vi "Fluids #4.vi"() -> ()   [LabVIEW 2017]
uses:
  <vilib>/addons/control/pid/pid.llb/PID Control Input Filter (DBL).vi
  <vilib>/addons/control/pid/pid.llb/PID Advanced (DBL).vi
  <vilib>/addons/control/pid/NI_PID_pid.lvlib
panel:
  in  "stop":bool
  in  "Pump Switch":bool
  out "Pump Delta P":dbl format="%.1f"
  out "Globe Valve Delta P":dbl format="%.1f"
  out "Ball Valve Delta P":dbl format="%.1f"
  out "EL Delta P":dbl format="%.1f"
  out "TEE Delta P":dbl format="%.1f"
  out "Pipe Delta P":dbl format="%.1f"
  out "U Delta P":dbl format="%.1f"
  out "Fluid Temperature":dbl=19.966648625034704 format="%.1f"
  in  "Flowrate Setpoint":dbl=10.0 caption="gal/min" format="%.1f"
  out "Liquid Flowrate":dbl=-2.4682881675745557e-11 format="%.1f"
  out "Control Valve":dbl(slide)=100.0 scale=0.0..100.0
  in  "Manual Control Override":bool=TRUE
  in  "Set Manual Valve Position":dbl(slide)=100.0 scale=0.0..100.0
  in  "Kc":dbl=2.0
  in  "Ti":dbl=0.05 caption="(min)"
  in  "Td":dbl caption="(min)"
  in  "Main Power":bool
  in  "Pump Speed Setpoint":dbl=100.0 caption="% of Nominal (3450 rpm)" min=0.0 max=125.0 format="%#.1f"
  out "Actual Pump Speed":dbl caption="RPM" format="%#.0f"
  out "Bypass Flowrate":dbl caption="gal/min" format="%#.1f"
  out "Bypass Delta P":dbl caption="psi" format="%#.1g"
  out "Pump Motor Power":dbl caption="W" format="%#.0f"
  out "Control Valve Delta P":dbl caption="psi" format="%#.1g"
  out "Data Point Count":i32
  in  "Specify Time between Data Points (sec)":dbl=1.0
  in  "Cancel Data Collection":bool
  in  "Specify number of data points":i16=1
  in  "Enable 3":bool
  out "Saving Data 3":bool
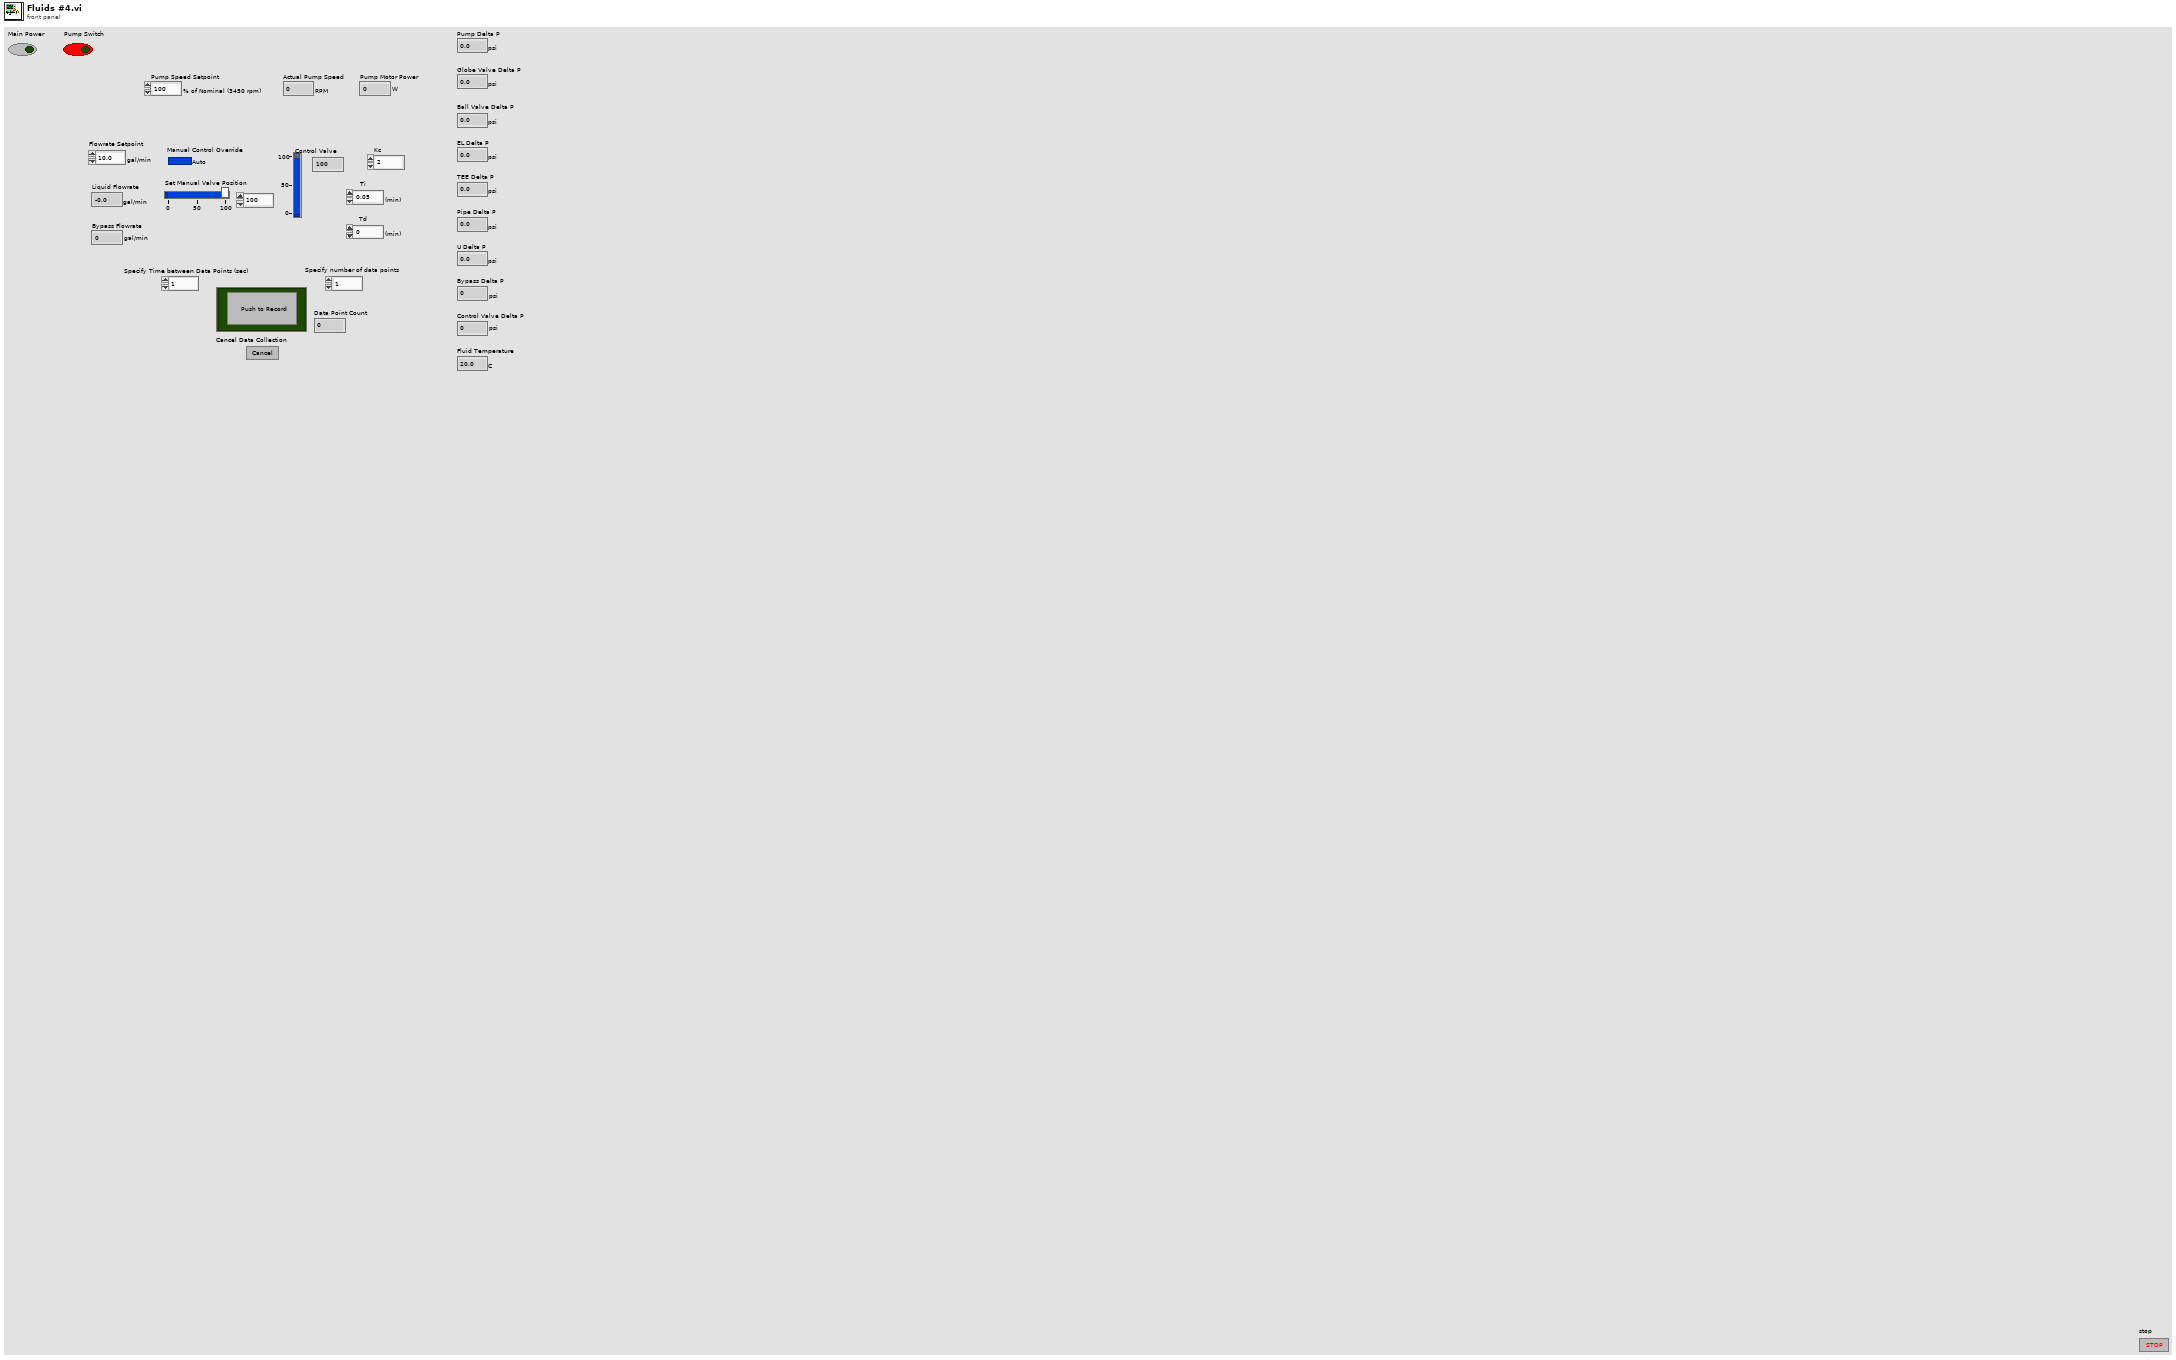
[diagram p1: front panel]
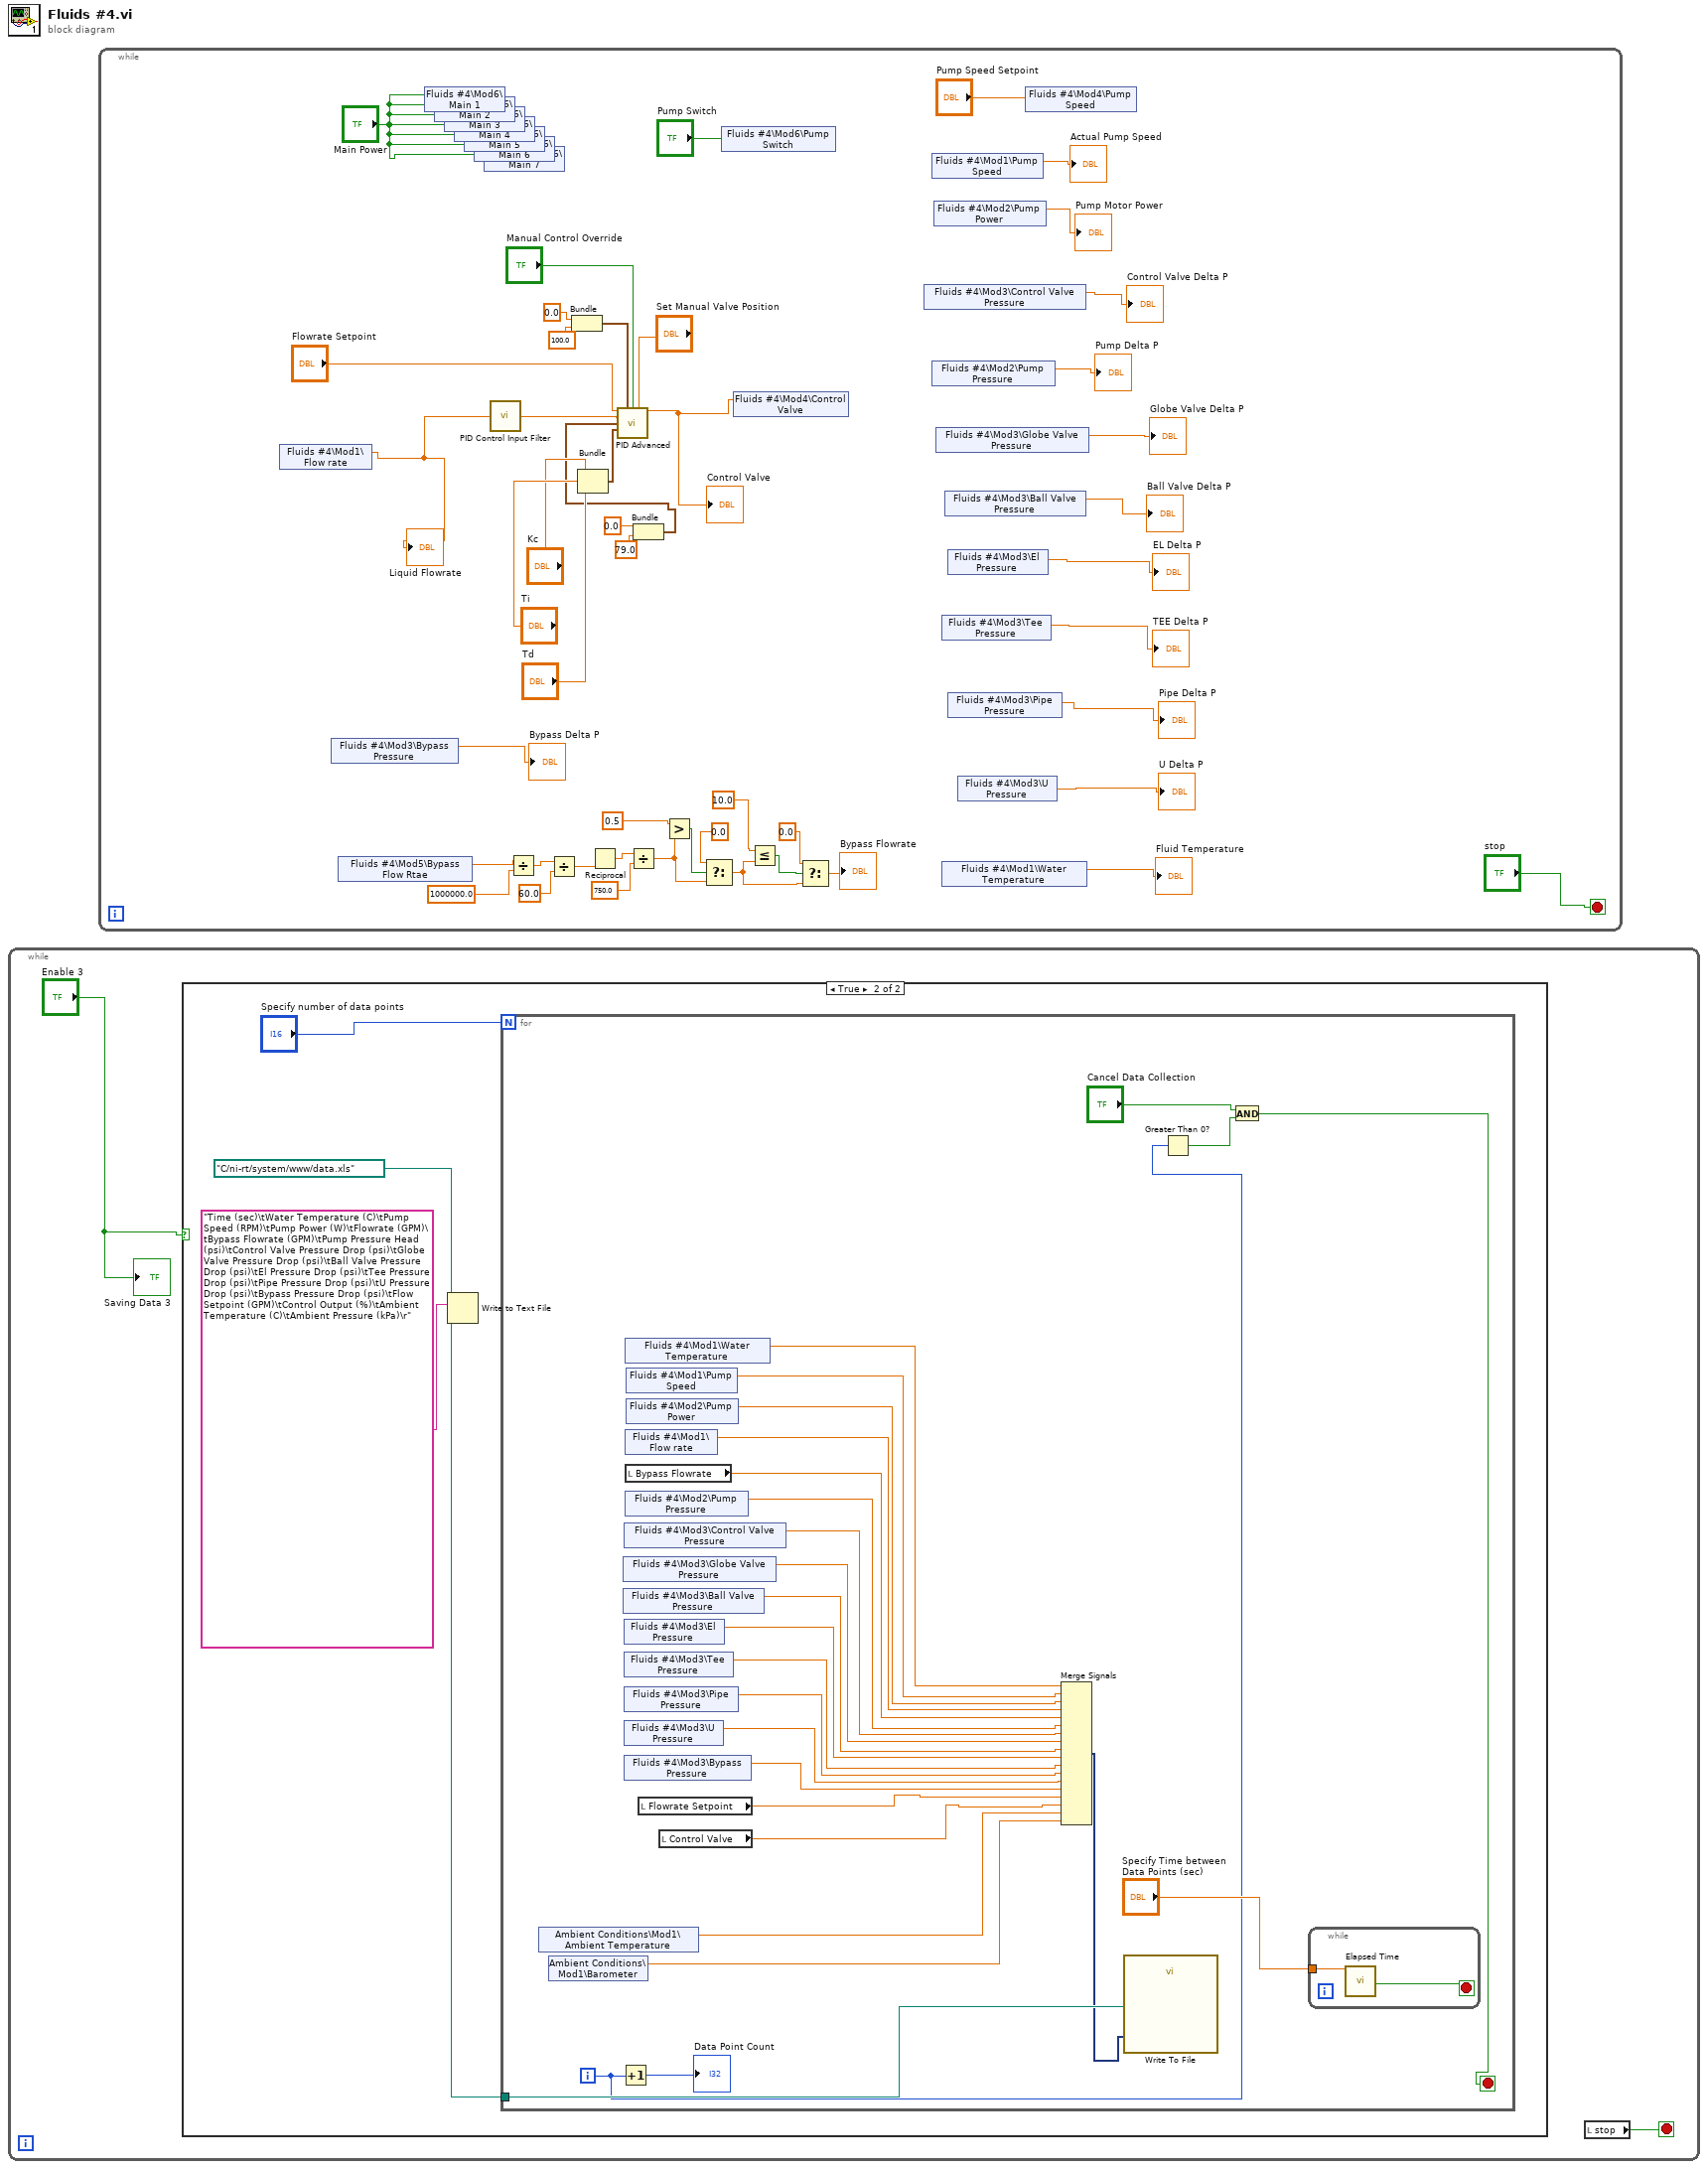
[diagram p0: block diagram]
diagram:
  n1 = while {
    stop <- w1 stop-if-true
    n2 = case shown="True" "Enable 3" {
      frame False {
      }
      frame True {
        w4 = path "C:/ni-rt/system/www/data.xls" ("Filename")
        n3 = Write to Text File(file (use dialog)=w4, text="Time (sec)\tWater Temperature (C)\tPump Speed (RPM)\tPump Power (W)\tFlowrate (GPM)\tBypass Flowrate (GPM)\tPump Pressure Head (psi)\tControl Valve Pressure Drop (psi)\tGlobe Valve Pressure Drop (psi)\tBall Valve Pressure Drop (psi)\tEl Pressure Drop (psi)\tTee Pressure Drop (psi)\tPipe Pressure Drop (psi)\tU Pressure Drop (psi)\tBypass Pressure Drop (psi)\tFlow Setpoint (GPM)\tControl Output (%)\tAmbient Temperature (C)\tAmbient Pressure (kPa)\r") -> ()  [unwired: 2 in, 3 out]
        n4 = for {
          N: "Specify number of data points" -> [_]
          tunnel: w4 -> [w31]
          i -> [w27]
          stop <- w24 stop-if-true
          n5 = shared-variable "Ambient Conditions\\Mod1\\Ambient Temperature"() -> (w23:dbl)  [unwired: 1 in, 1 out]
          n6 = shared-variable "Ambient Conditions\\Mod1\\Barometer"() -> (w22:dbl)  [unwired: 1 in, 1 out]
          n7 = Increment(x=w27) -> (x+1=→"Data Point Count":i32)
          n8 = shared-variable "Fluids #4\\Mod3\\Globe Valve Pressure"() -> (w15:dbl)  [unwired: 1 in, 1 out]
          n9 = shared-variable "Fluids #4\\Mod3\\Ball Valve Pressure"() -> (w16:dbl)  [unwired: 1 in, 1 out]
          n10 = shared-variable "Fluids #4\\Mod3\\Control Valve Pressure"() -> (w14:dbl)  [unwired: 1 in, 1 out]
          n11 = shared-variable "Fluids #4\\Mod3\\El Pressure"() -> (w17:dbl)  [unwired: 1 in, 1 out]
          n12 = shared-variable "Fluids #4\\Mod3\\Tee Pressure"() -> (w18:dbl)  [unwired: 1 in, 1 out]
          n13 = shared-variable "Fluids #4\\Mod3\\Pipe Pressure"() -> (w19:dbl)  [unwired: 1 in, 1 out]
          n14 = shared-variable "Fluids #4\\Mod3\\U Pressure"() -> (w20:dbl)  [unwired: 1 in, 1 out]
          n15 = shared-variable "Fluids #4\\Mod3\\Bypass Pressure"() -> (w21:dbl)  [unwired: 1 in, 1 out]
          n16 = shared-variable "Fluids #4\\Mod1\\Water Temperature"() -> (w9:dbl)  [unwired: 1 in, 1 out]
          n17 = shared-variable "Fluids #4\\Mod1\\Flow rate"() -> (w12:dbl)  [unwired: 1 in, 1 out]
          n18 = local read "Bypass Flowrate"() -> (w6:dbl)
          n19 = shared-variable "Fluids #4\\Mod2\\Pump Pressure"() -> (w13:dbl)  [unwired: 1 in, 1 out]
          n20 = shared-variable "Fluids #4\\Mod1\\Pump Speed"() -> (w10:dbl)  [unwired: 1 in, 1 out]
          n21 = shared-variable "Fluids #4\\Mod2\\Pump Power"() -> (w11:dbl)  [unwired: 1 in, 1 out]
          n22 = local read "Flowrate Setpoint"() -> (w8:dbl)
          n23 = local read "Control Valve"() -> (w7:dbl)
          n24 = Merge Signals(w9, w10, w11, w12, w6, w13, w14, w15, w16, w17, w18, w19, w20, w21, w8, w7, w23, w22) -> (w29:dynamicdata)
          n25 = call "Write To File"("Signals"=w29, "Filename"=w31) -> ()  [unwired: 15 in, 3 out]
          n26 = Greater Than 0?(x=w27) -> (x > 0?=w25:bool)
          n27 = And(x="Cancel Data Collection", y=w25) -> (x .and. y?=w24:bool)
          n28 = while {
            tunnel: "Specify Time between Data Points (sec)" -> [w32]
            stop <- w33 stop-if-true
            n29 = call "Elapsed Time"("Time Target (s)"=w32) -> ("Time has Elapsed"=w33:bool)  [unwired: 11 in, 7 out]
          }
        }
      }
    }
    n30 = local read "stop"() -> (w1:bool)
    "Saving Data 3" <- "Enable 3"
  }
  n31 = while {
    stop <- "stop" stop-if-true
    n32 = shared-variable "Fluids #4\\Mod1\\Flow rate"() -> (w62:dbl)  [unwired: 1 in, 1 out]
    "Liquid Flowrate" <- w62
    n33 = shared-variable "Fluids #4\\Mod3\\Bypass Pressure"() -> (→"Bypass Delta P":dbl)  [unwired: 1 in, 1 out]
    n34 = shared-variable "Fluids #4\\Mod5\\Bypass Flow Rtae"() -> (w52:dbl)  [unwired: 1 in, 1 out]
    n35 = shared-variable "Fluids #4\\Mod6\\Main 1"("Main Power") -> ()  [unwired: 1 in, 1 out]
    n36 = shared-variable "Fluids #4\\Mod6\\Main 2"("Main Power") -> ()  [unwired: 1 in, 1 out]
    n37 = shared-variable "Fluids #4\\Mod6\\Main 3"("Main Power") -> ()  [unwired: 1 in, 1 out]
    n38 = shared-variable "Fluids #4\\Mod6\\Main 4"("Main Power") -> ()  [unwired: 1 in, 1 out]
    n39 = shared-variable "Fluids #4\\Mod6\\Main 5"("Main Power") -> ()  [unwired: 1 in, 1 out]
    n40 = shared-variable "Fluids #4\\Mod6\\Main 6"("Main Power") -> ()  [unwired: 1 in, 1 out]
    n41 = shared-variable "Fluids #4\\Mod6\\Main 7"("Main Power") -> ()  [unwired: 1 in, 1 out]
    n42 = call-poly <vilib>:"PID Control Input Filter.vi"("input"=w62) -> ("output"=w68:dbl)  [unwired: 4 in]
    n43 = Divide(x=w52, y=1000000.0) -> (x/y=w50:dbl)
    n44 = Divide(x=w50, y=60.0) -> (x/y=w48:dbl)
    n45 = Bundle(0.0, 100.0) -> (w70:cluster{dbl, dbl})  [unwired: 1 in]
    n46 = Bundle("Kc"="Kc", "Ti"="Ti", "Td"="Td") -> (w80:cluster{"Kc":dbl, "Ti":dbl, "Td":dbl})  [unwired: 1 in]
    n47 = Reciprocal(x=w48) -> (1/x=w47:dbl)
    n48 = Divide(x=w47, y=750.0) -> (x/y=w44:dbl)
    n49 = Bundle(0.0, 79.0) -> (w74:cluster{dbl, dbl})  [unwired: 1 in]
    n50 = call-poly <vilib>:"PID Advanced.vi"("setpoint"="Flowrate Setpoint", "output range"=w70, "auto? (T)"="Manual Control Override", "manual control"="Set Manual Valve Position", "process variable"=w68, "setpoint range"=w74, "PID gains"=w80) -> ("output"=w35:dbl)  [unwired: 7 in, 1 out]
    "Control Valve" <- w35
    n51 = Greater?(x=0.5, y=w44) -> (0:w42:bool)
    n52 = Select(t=0.0, s=w42, f=w44) -> (s? t:f=w41:dbl)
    n53 = shared-variable "Fluids #4\\Mod6\\Pump Switch"("Pump Switch") -> ()  [unwired: 1 in, 1 out]
    n54 = shared-variable "Fluids #4\\Mod4\\Control Valve"(w35) -> ()  [unwired: 1 in, 1 out]
    n55 = Less Or Equal?(x=10.0, y=w41) -> (x <= y?=w39:bool)
    n56 = Select(t=0.0, s=w39, f=w41) -> (s? t:f=→"Bypass Flowrate":dbl)
    n57 = shared-variable "Fluids #4\\Mod3\\Control Valve Pressure"() -> (→"Control Valve Delta P":dbl)  [unwired: 1 in, 1 out]
    n58 = shared-variable "Fluids #4\\Mod1\\Pump Speed"() -> (→"Actual Pump Speed":dbl)  [unwired: 1 in, 1 out]
    n59 = shared-variable "Fluids #4\\Mod2\\Pump Pressure"() -> (→"Pump Delta P":dbl)  [unwired: 1 in, 1 out]
    n60 = shared-variable "Fluids #4\\Mod2\\Pump Power"() -> (→"Pump Motor Power":dbl)  [unwired: 1 in, 1 out]
    n61 = shared-variable "Fluids #4\\Mod3\\Globe Valve Pressure"() -> (→"Globe Valve Delta P":dbl)  [unwired: 1 in, 1 out]
    n62 = shared-variable "Fluids #4\\Mod3\\Tee Pressure"() -> (→"TEE Delta P":dbl)  [unwired: 1 in, 1 out]
    n63 = shared-variable "Fluids #4\\Mod1\\Water Temperature"() -> (→"Fluid Temperature":dbl)  [unwired: 1 in, 1 out]
    n64 = shared-variable "Fluids #4\\Mod3\\Ball Valve Pressure"() -> (→"Ball Valve Delta P":dbl)  [unwired: 1 in, 1 out]
    n65 = shared-variable "Fluids #4\\Mod3\\El Pressure"() -> (→"EL Delta P":dbl)  [unwired: 1 in, 1 out]
    n66 = shared-variable "Fluids #4\\Mod3\\Pipe Pressure"() -> (→"Pipe Delta P":dbl)  [unwired: 1 in, 1 out]
    n67 = shared-variable "Fluids #4\\Mod3\\U Pressure"() -> (→"U Delta P":dbl)  [unwired: 1 in, 1 out]
    n68 = shared-variable "Fluids #4\\Mod4\\Pump Speed"("Pump Speed Setpoint") -> ()  [unwired: 1 in, 1 out]
  }
